vi "Launch [V] Login.vi"(8 "error in (no error)":errorcluster, 11 "[C] User Management in":refnum<class "[C] User Management.lvclass">) -> (0 "error out":errorcluster, 3 "[C] User Management out":refnum<class "[C] User Management.lvclass">)   [LabVIEW 2020, in "[C] User Management.lvlib" / "[C] User Management.lvclass"]
uses:
  [C] User Management.lvclass
  [V] Login/[V] Login/[V] Login.lvclass
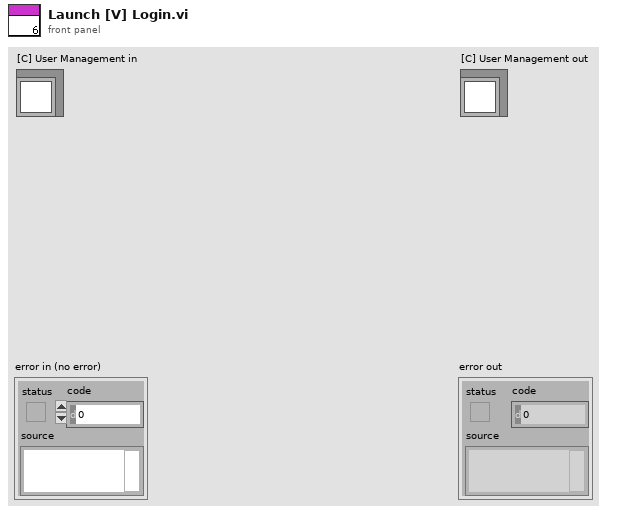
[diagram p1: front panel]
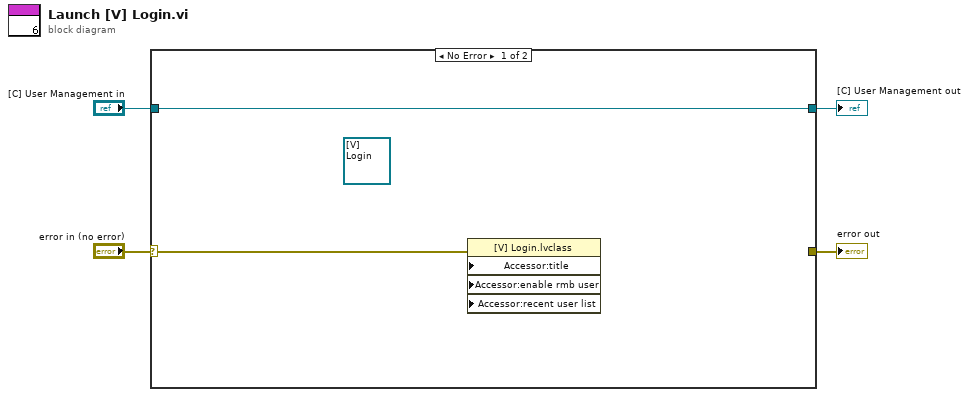
[diagram p0: block diagram]
diagram:
  n1 = case shown="No Error" "error in (no error)" {
    selector: "error in (no error)" -> [w5 w8]
    tunnel: [_ w8] -> w3
    tunnel: [w6 w7] -> w1
    tunnel: "[C] User Management in" -> [w6 w7]
    frame No Error {
      (unwired) refnum<class "[V] Login.lvclass"> refnum ("[V] Login.lvlib:[V] Login.lvclass")
      n2 = property class="[V] Login.lvclass" props=["Accessor:title", "Accessor:enable rmb user", "Accessor:recent user list"](error in=w5) -> ()  [unwired: 4 in, 2 out]
    }
    frame Error {
    }
  }
  "error out" <- w3
  "[C] User Management out" <- w1
